vi "PH_ImageOperator.write PSDB Beam Analysis data.vi"(0 "i ref in":refnum<vi>, 5 "error in":errorcluster) -> (14 "i ref out":refnum<vi>, 16 "BA Boolean data":T3[](array[typedef]), 17 "BA Numeric data":T2[](array[typedef]), 18 "BA String data":T1[](array[typedef]), 19 "error out":errorcluster)   [LabVIEW 2014, in "PH_ImageOperator.lvlib"]
uses:
  PH_ImageOperator.lvlib
  PH_PSDBWriter/PH_PSDBWriter.Boolean dataset.ctl
  PH_PSDBWriter/PH_PSDBWriter.Numeric dataset.ctl
  PH_PSDBWriter/PH_PSDBWriter.String dataset.ctl
  PH_StatusHandler/PH_StatusHandler.Status.ctl
  PH_PSDBWriter/PH_PSDBWriter.lvlib
  PH_StatusHandler/PH_StatusHandler.lvlib
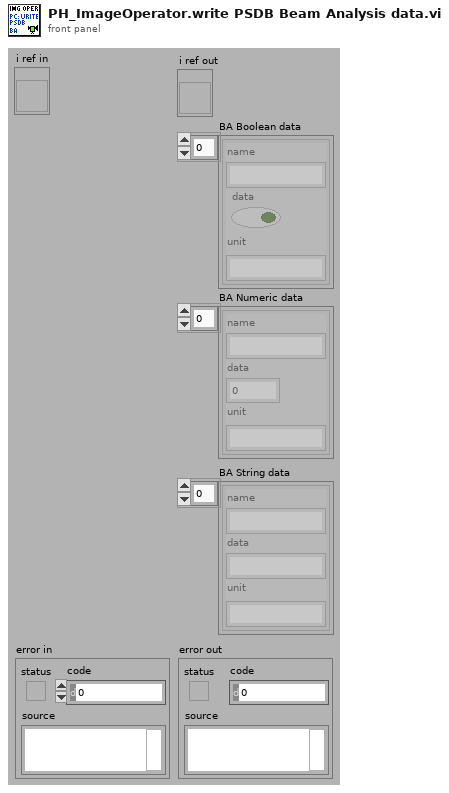
[diagram p1: front panel]
types:
  T1 = typedef "PH_PSDBWriter.lvlib/PH_PSDBWriter.String dataset.ctl" = cluster{"name":string, "data":string, "unit":string}
  T2 = typedef "PH_PSDBWriter.lvlib/PH_PSDBWriter.Numeric dataset.ctl" = cluster{"name":string, "data":dbl, "unit":string}
  T3 = typedef "PH_PSDBWriter.lvlib/PH_PSDBWriter.Boolean dataset.ctl" = cluster{"name":string, "data":bool, "unit":string}
  T4 = typedef "PH_ImageOperator.lvlib/PH_ImageOperator.i attribute.ctl" = cluster{"GUI Refs":cluster{"Delete":refnum<vi>, "Calibration status":refnum<vi>, "BI subtracted":refnum<vi>, "calc Energy":refnum<vi>, "Energy: expected value":refnum<vi>, "Energy: Tolerance":refnum<vi>, "Energy calculated":refnum<vi>, "Energy":refnum<vi>, "calc Beam Anal":refnum<vi>, "Maj Diam 1/esquare":refnum<vi>, "Min Diam 1/esquare":refnum<vi>, "Azi Angle":refnum<vi>, "Min/Maj Diam esquare":refnum<vi>, "Beam analysed":refnum<vi>, "CoG - x":refnum<vi>, "CoG - y":refnum<vi>, "BA: Method":refnum<vi>, "BA: Steps":refnum<vi>, "BA: Factor":refnum<vi>, "calc Traces":refnum<vi>, "Traces: Fit Gauss":refnum<vi>, "Traces calculated":refnum<vi>, "Maj FWHM":refnum<vi>, "Min FWHM":refnum<vi>, "Major Trace":refnum<vi>, "Minor Trace":refnum<vi>, "Maj Fit Order":refnum<vi>, "Min Fit Order":refnum<vi>, "Position calculated":refnum<vi>, "Position":refnum<vi>, "Type":refnum<vi>, "Center":refnum<vi>, "exp - X":refnum<vi>, "exp - Y":refnum<vi>, "Tolerance":refnum<vi>, "f":refnum<vi>, "M":refnum<vi>, "D":refnum<vi>, "q":refnum<vi>, "Dummy Method":refnum<vi>, "Dummy Type":refnum<vi>, "Global On":refnum<vi>, "Traces: No offset":refnum<vi>, "Maj 99%":refnum<vi>, "Min 99%":refnum<vi>, "GUI FF Image":refnum<vi>, "calc Fill Factor":refnum<vi>, "FF calculated":refnum<vi>, "Fill Factor: Filter?":refnum<vi>, "FF: Damage Threshold":refnum<vi>, "FF: Threshold":refnum<vi>, "FF: max allow. Energy":refnum<vi>, "FF: Fillfactor":refnum<vi>, "Calibration data":refnum<vi>}, "List of GUIs":string[], "Calibration":cluster{"Status":T5, "Calibration data":T6, "Calibration Data File":path}, "Final Image":cluster{"BI Subtraction Failure":bool}, "Energy":cluster{"on":bool, "expected value [mJ]":dbl, "Tolerance [%]":dbl, "State":T5, "Energy [mJ]":dbl, "Unit":string, "calculated @":timestamp}, "Beam Analysis":cluster{"on":bool, "Data":T7, "Method":bool, "Steps":i32, "Factor":i32, "ROI":cluster{"Left":i32, "Top":i32, "Right":i32, "Bottom":i32}, "analysed @":timestamp}, "Trace Analysis":cluster{"on":bool, "Fit on":bool, "Maj FWHM":dbl, "Min FWHM":dbl, "Maj Fit Order":i32, "Min Fit Order":i32, "No Offset":bool, "Maj 99%":dbl, "Min 99%":dbl, "Traces":cluster{"XScaleName":string, "Y Scale Minimum":sgl, "Y Scale Maximum":sgl, "X Scale Minimum":sgl, "X Scale Maximum":sgl, "Traces":cluster{"Index":sgl[], "Trace":dbl[]}[]}[], "analysed @":timestamp}, "Position Analysis":cluster{"on":bool, "exp - X":i32, "exp - Y":i32, "focal length [mm]":dbl, "Magnification":dbl, "Delta":dbl, "Theta":dbl, "Tolerance":dbl, "Type":bool, "analysed @":timestamp}, "Fill Factor":cluster{"on":bool, "Filter on?":bool, "Threshold":dbl, "Damage Threshold [J/cm²]":dbl, "Fillfactor":dbl, "Max. allowed Energy [J]":dbl, "calculated @":timestamp}, "Statistician Service ID":i32, "Images":cluster{"Background":T8, "OP":T8, "GUI":T8, "BA: ROI":T8, "Trace: Turn":T8, "FF: Main":T8, "FF: Help":T8, "PSDB: BG":T8, "PSDB: OP":T8, "PSDB: FF":T8}}
  T5 = typedef "PH_StatusHandler.lvlib/PH_StatusHandler.Status.ctl" = i16
  T6 = typedef "PH_ImageCalibrator.lvlib/PH_ImageCalibrator.Calibration Data.ctl" = cluster{"Date":string, "Time":string, "Cam Settings":cluster{"Cam ID":string, "Gain":dbl, "Brightness":dbl, "Shutter":dbl, "Cam Error":bool, "Mode":i32}, "Background Image":cluster{"Image":dbl[][], "Image Error":bool}, "Linear Calibration":cluster{"Calibration Factor":dbl, "not mm or mrad":bool}, "Energy Calibration":cluster{"Calibration Factor":dbl, "no mJ":bool}}
  T7 = typedef "PH_ImageOperator.lvlib/PH_ImageOperator.Beam Analysis Data.ctl" = cluster{"CoG-x":sgl, "CoG-y":sgl, "Maj Dim":dbl, "Min Dim":dbl, "Ellipticity":dbl, "Azimuth Angle [rad]":dbl, "Azi Angle rel to Maj?":bool}
  T8 = typedef "IMAQ Image.ctl" = refnum<image>
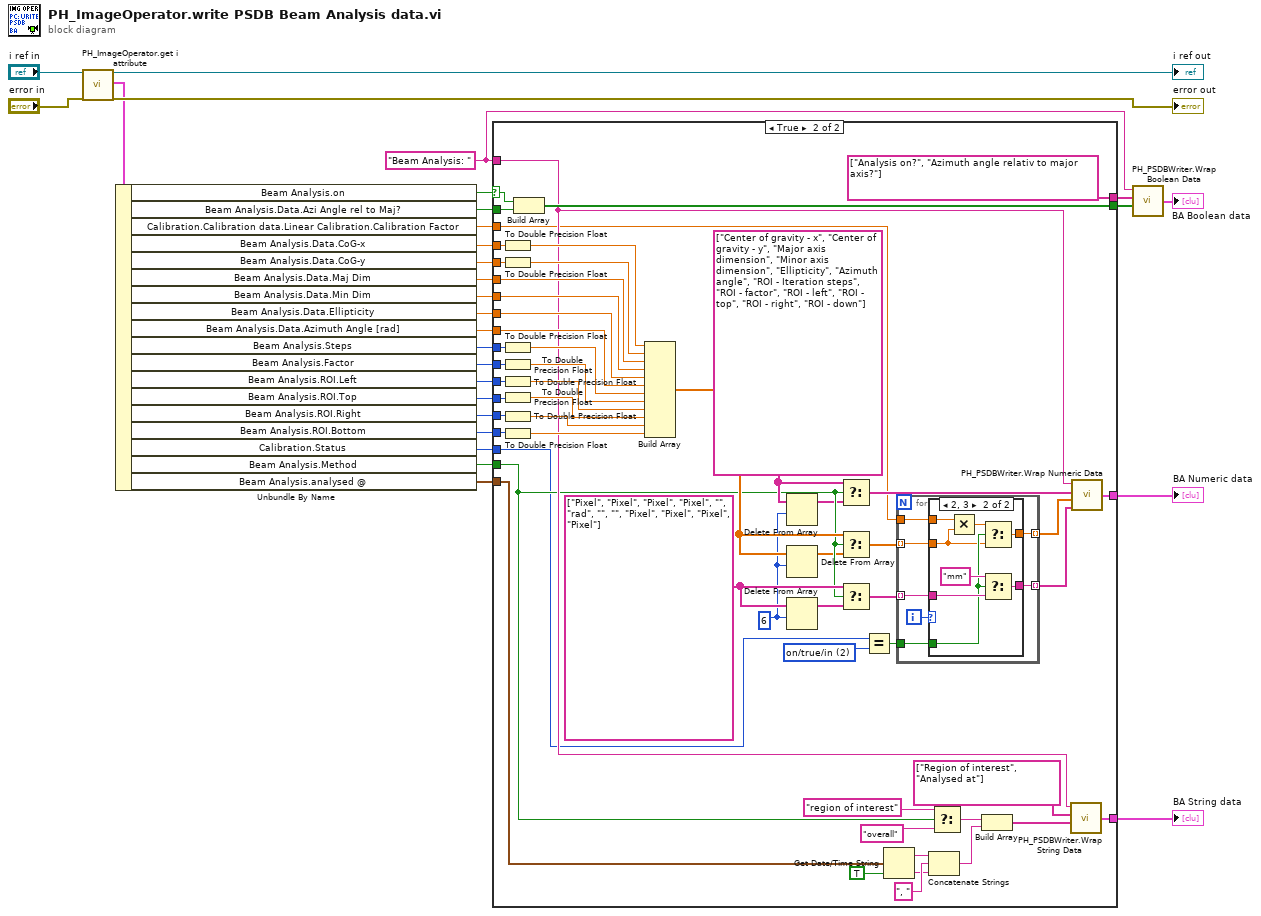
[diagram p0: block diagram]
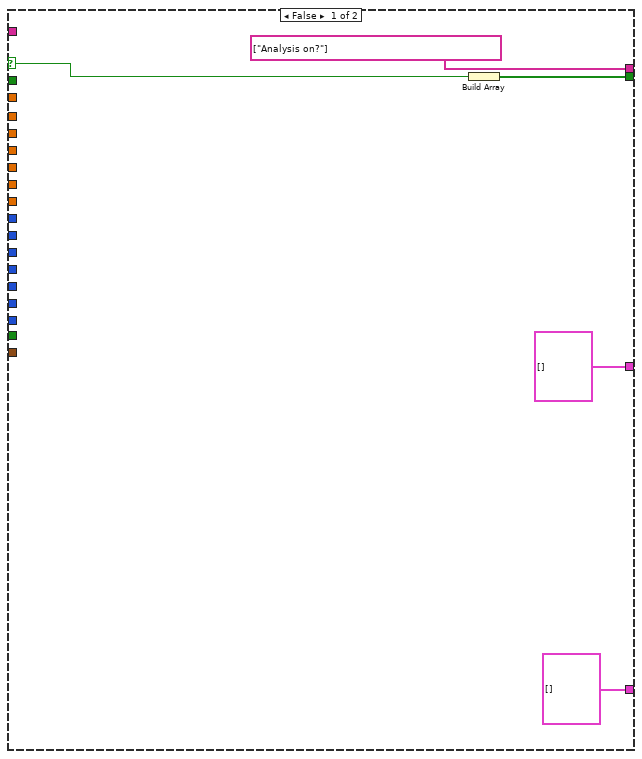
[diagram p2: hidden frame]
diagram:
  w3 = "Beam Analysis: " ("string")
  n1 = call "PH_ImageOperator.get i attribute.vi"("i ref in"="i ref in", "error in (no error)"="error in") -> ("i ref out"=→"i ref out":refnum<vi>, "i attribute"=w24:T4, "error out"=→"error out":errorcluster)  [unwired: 15 in]
  n2 = Unbundle By Name(w24) -> ("Beam Analysis.on"=w7:bool, "Beam Analysis.Data.Azi Angle rel to Maj?"=w23:bool, "Calibration.Calibration data.Linear Calibration.Calibration Factor"=w1:dbl, "Beam Analysis.Data.CoG-x"=w17:sgl, "Beam Analysis.Data.CoG-y"=w18:sgl, "Beam Analysis.Data.Maj Dim"=w22:dbl, "Beam Analysis.Data.Min Dim"=w21:dbl, "Beam Analysis.Data.Ellipticity"=w20:dbl, "Beam Analysis.Data.Azimuth Angle [rad]"=w19:dbl, "Beam Analysis.Steps"=w16:i32, "Beam Analysis.Factor"=w15:i32, "Beam Analysis.ROI.Left"=w13:i32, "Beam Analysis.ROI.Top"=w12:i32, "Beam Analysis.ROI.Right"=w11:i32, "Beam Analysis.ROI.Bottom"=w10:i32, "Calibration.Status"=w9:T5, "Beam Analysis.Method"=w8:bool, "Beam Analysis.analysed @"=w6:timestamp)
  n3 = case shown="True" w7 {
    selector: w7 -> [w31 w59]
    tunnel: [T2[] [] w50] -> w25
    tunnel: w23 -> [_ w58]
    tunnel: w22 -> [_ w87]
    tunnel: w21 -> [_ w86]
    tunnel: w20 -> [_ w85]
    tunnel: w19 -> [_ w84]
    tunnel: w18 -> [_ w83]
    tunnel: w17 -> [_ w81]
    tunnel: w16 -> [_ w79]
    tunnel: w15 -> [_ w78]
    tunnel: [T1[] [] w54] -> w14
    tunnel: w13 -> [_ w75]
    tunnel: w12 -> [_ w74]
    tunnel: w11 -> [_ w73]
    tunnel: w10 -> [_ w72]
    tunnel: w9 -> [_ w38]
    tunnel: w8 -> [_ w40]
    tunnel: w6 -> [_ w66]
    tunnel: w3 -> [_ w52]
    tunnel: [w30 w57] -> w5
    tunnel: [string[] ["Analysis on?"] string[] ["Analysis on?", "Azimuth angle relativ to major axis?"]] -> w4
    tunnel: w1 -> [_ w39]
    frame False {
      n4 = Build Array(w31) -> (w30:bool[])
    }
    frame True {
      w42 = string[] ["Pixel", "Pixel", "Pixel", "Pixel", "", "rad", "", "", "Pixel", "Pixel", "Pixel", "Pixel"]
      w41 = 6 ("length")
      w48 = string[] ["Center of gravity - x", "Center of gravity - y", "Major axis dimension", "Minor axis dimension", "Ellipticity", "Azimuth angle", "ROI - Iteration steps", "ROI - factor", "ROI - left", "ROI - top", "ROI - right", "ROI - down"]
      w67 = T5 2 items=["no info", "off/false/out", "on/true/in", "Failure", "Alarm", "Status 1", "Status 2", "Status 3"] ("Calibration.Status")
      n5 = To Double Precision Float(number=w81) -> (double precision float=w80:dbl)
      n6 = To Double Precision Float(number=w83) -> (double precision float=w82:dbl)
      n7 = To Double Precision Float(number=w79) -> (double precision float=w77:dbl)
      n8 = To Double Precision Float(number=w78) -> (double precision float=w76:dbl)
      n9 = To Double Precision Float(number=w75) -> (double precision float=w71:dbl)
      n10 = To Double Precision Float(number=w74) -> (double precision float=w70:dbl)
      n11 = To Double Precision Float(number=w73) -> (double precision float=w69:dbl)
      n12 = To Double Precision Float(number=w72) -> (double precision float=w68:dbl)
      n13 = Build Array(w59, w58) -> (w57:bool[])
      n14 = Build Array(w80, w82, w87, w86, w85, w84, w77, w76, w71, w70, w69, w68) -> (w49:dbl[])
      n15 = Delete From Array(array=w48, length=w41) -> (array with subset deleted=w37:string[])  [unwired: 1 in, 1 out]
      n16 = Delete From Array(array=w49, length=w41) -> (array with subset deleted=w36:dbl[])  [unwired: 1 in, 1 out]
      n17 = Delete From Array(array=w42, length=w41) -> (array with subset deleted=w35:string[])  [unwired: 1 in, 1 out]
      n18 = Select(t=w48, s=w40, f=w37) -> (s? t:f=w51:string[])
      n19 = Select(t=w49, s=w40, f=w36) -> (s? t:f=w47:dbl[])
      n20 = Select(t=w42, s=w40, f=w35) -> (s? t:f=w43:string[])
      n21 = Equal?(x=w38, y=w67) -> (x = y?=w44:bool)
      n22 = Get Date/Time String(seconds (now)=w66, want seconds? (F)=TRUE) -> (date string=w64:string, time string=w62:string)  [unwired: 1 in]
      n23 = for {
        tunnel: [w95] -> w46 mode=indexing
        tunnel: w47 -> [w96] mode=indexing
        tunnel: w43 -> [w94] mode=indexing
        tunnel: [w93] -> w45 mode=indexing
        tunnel: w44 -> [w91]
        tunnel: w39 -> [w90]
        i -> [w92]
        n24 = case shown="2, 3" w92 {
          tunnel: w96 -> [w98 w101]
          tunnel: [w98 w103] -> w95
          tunnel: w94 -> [w97 w106]
          tunnel: [w97 w105] -> w93
          tunnel: w91 -> [_ w102]
          tunnel: w90 -> [_ w99]
          frame Default {
          }
          frame 2, 3 {
            n25 = Multiply(x=w99, y=w101) -> (x*y=w100:dbl)
            n26 = Select(t=w100, s=w102, f=w101) -> (s? t:f=w103:dbl)
            n27 = Select(t="mm", s=w102, f=w106) -> (s? t:f=w105:string)
          }
        }
      }
      n28 = Concatenate Strings(w64, ", " ("string"), w62) -> (w61:string)
      n29 = Select(t="region of interest", s=w40, f="overall" ("string")) -> (s? t:f=w60:string)
      n30 = Build Array(w60, w61) -> (w55:string[])
      n31 = call "PH_PSDBWriter.Wrap String Data.vi"("Data Array"=w55, "Name Array"=string[] ["Region of interest", "Analysed at"], "Name Prefix"=w52) -> ("PSDB String Data Array"=w54:T1[])  [unwired: 1 in]
      n32 = call "PH_PSDBWriter.Wrap Numeric Data.vi"("Unit Array"=w45, "Data Array"=w46, "Name Array"=w51, "Name Prefix"=w52) -> ("PSDB Numeric Data Array"=w50:T2[])
    }
  }
  "BA Numeric data" <- w25
  "BA String data" <- w14
  n33 = call "PH_PSDBWriter.Wrap Boolean Data.vi"("Data Array"=w5, "Name Array"=w4, "Name Prefix"=w3) -> ("PSDB Boolean Data Array"=→"BA Boolean data":T3[])  [unwired: 1 in]
